vi "Read Version.vi"(8 "error in (no error)":errorcluster, 11 "Simple Build GUI in":refnum<class "Simple Build GUI.lvclass">) -> (0 "error out":errorcluster, 3 "Simple Build GUI out":refnum<class "Simple Build GUI.lvclass">)   [LabVIEW 2020, in "Builder Tools.lvlib" / "Simple Build GUI.lvclass"]
uses:
  Simple Build GUI.lvclass
  Simple Build GUI.lvclass/Simple Build GUI.ctl
  Builder/Builder.lvclass
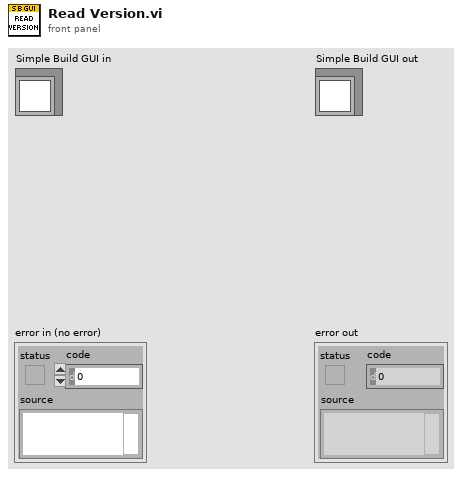
[diagram p1: front panel]
types:
  T1 = typedef "Builder Core.lvlib/Version.ctl" = cluster{"Major":u16, "Minor":u16, "Fix":u16, "Build":u16}
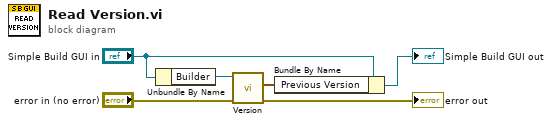
[diagram p0: block diagram]
diagram:
  n1 = Unbundle By Name("Simple Build GUI in") -> ("Builder"=w5:refnum<class "Builder.lvclass">)
  n2 = call "Version.vi"("error in (no error)"="error in (no error)", "Builder in"=w5) -> ("error out"=→"error out":errorcluster, "Version"=w1:T1)  [unwired: 7 in, 1 out]
  n3 = Bundle By Name(cluster="Simple Build GUI in", "Previous Version"=w1) -> (→"Simple Build GUI out":refnum<class "Simple Build GUI.lvclass">)
